vi "json_array.vi"(7 "indent level":i32, 10 "Array of JSON Elements":string[](array[string]), 11 "name":string) -> (3 "indented string":string)   [LabVIEW 2013, in "Caraya.lvlib" / "Test Result.lvclass"]
uses:
  Test Result.lvclass
  <vilib>/Utility/error.llb/whitespace.ctl
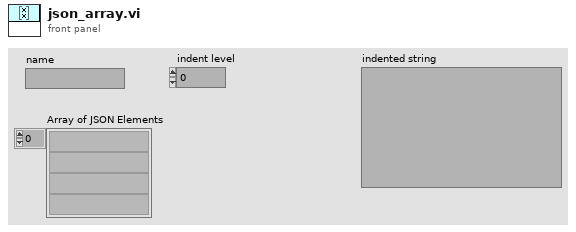
[diagram p1: front panel]
types:
  T1 = typedef "whitespace.ctl" = u16
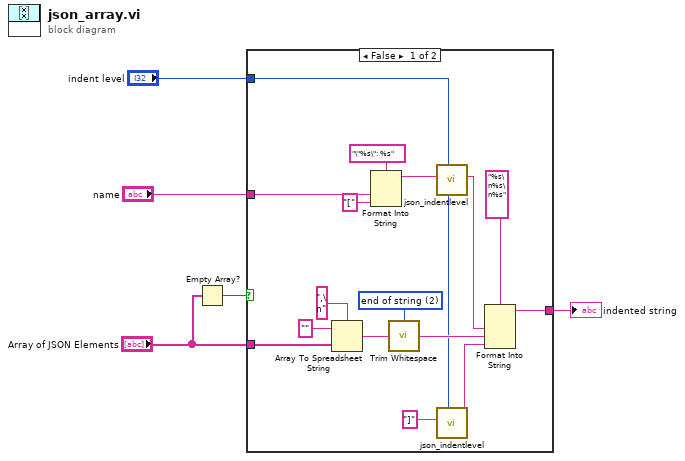
[diagram p0: block diagram]
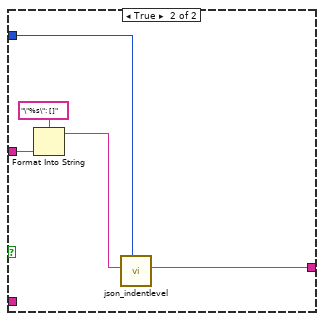
[diagram p2: hidden frame]
diagram:
  n1 = Empty Array?(array="Array of JSON Elements") -> (empty?=w4:bool)
  n2 = case shown="False" w4 {
    tunnel: "Array of JSON Elements" -> [w6 _]
    tunnel: [w16 w23] -> w1
    tunnel: "name" -> [w10 w25]
    tunnel: "indent level" -> [w7 w24]
    frame False {
      w19 = T1 2 items=["both", "start of string", "end of string"] ("location (both)")
      n3 = Array To Spreadsheet String(delimiter (Tab)=",\n", array=w6, 3:"" ("format string")) -> (spreadsheet string=w18:string)
      n4 = Format Into String(format string="\"%s\": %s", w10, "[" ("format string")) -> (resulting string=w11:string)  [unwired: 2 in, 1 out]
      n5 = call <vilib>:"Trim Whitespace.vi"("string"=w18, "location (both)"=w19) -> ("trimmed string"=w15:string)
      n6 = call "json_indentlevel.vi"("indent level"=w7, "string"=w11) -> ("indented string"=w14:string)  [unwired: 9 in]
      n7 = call "json_indentlevel.vi"("indent level"=w7, "string"="]" ("format string")) -> ("indented string"=w13:string)  [unwired: 9 in]
      n8 = Format Into String(format string="%s\n%s\n%s", w14, w15, w13) -> (resulting string=w16:string)  [unwired: 2 in, 1 out]
    }
    frame True {
      n9 = Format Into String(format string="\"%s\": []", w25) -> (resulting string=w26:string)  [unwired: 2 in, 1 out]
      n10 = call "json_indentlevel.vi"("indent level"=w24, "string"=w26) -> ("indented string"=w23:string)  [unwired: 9 in]
    }
  }
  "indented string" <- w1
